vi "Write Roles.vi"(8 "error in (no error)":errorcluster, 10 "Roles":T1, 11 "KickoffEnemyPlayVSS in":refnum<class "KickoffEnemyPlayVSS.lvclass">) -> (0 "error out":errorcluster, 3 "KickoffEnemyPlayVSS out":refnum<class "KickoffEnemyPlayVSS.lvclass">)   [LabVIEW 2020, in "KickoffEnemyPlayVSS.lvclass"]
uses:
  KickoffEnemyPlayVSS.lvclass
  NormalAttackerRoleVSS_class/NormalAttackerRoleVSS.lvclass
  KeeperRoleVSS_class/KeeperRoleVSS.lvclass
  DefenderAreaRoleVSS_class/DefenderAreaRoleVSS.lvclass
  KickoffEnemyPlayVSS.lvclass/KickoffEnemyPlayVSS.ctl
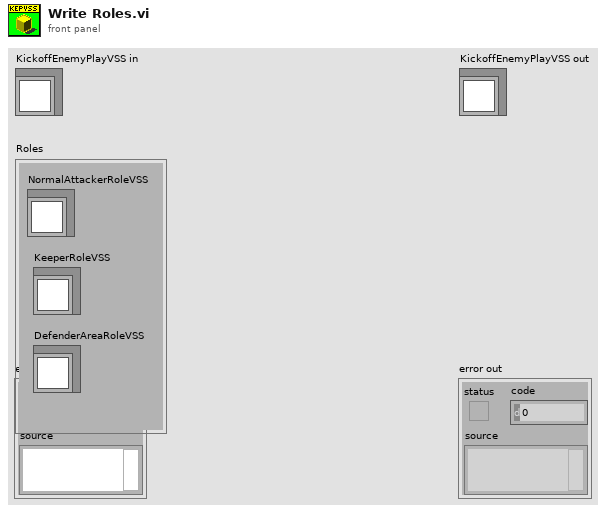
[diagram p1: front panel]
types:
  T1 = cluster{"NormalAttackerRoleVSS":refnum<class "NormalAttackerRoleVSS.lvclass">, "KeeperRoleVSS":refnum<class "KeeperRoleVSS.lvclass">, "DefenderAreaRoleVSS":refnum<class "DefenderAreaRoleVSS.lvclass">}
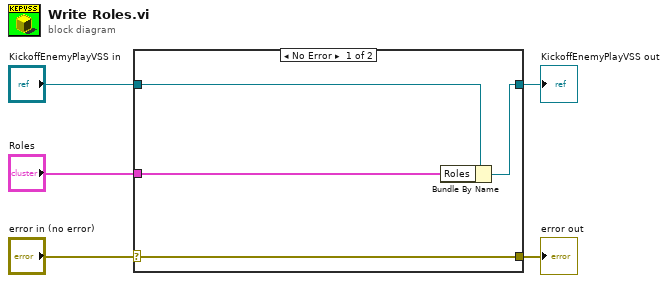
[diagram p0: block diagram]
diagram:
  n1 = case shown="No Error" "error in (no error)" {
    selector: "error in (no error)" -> [w9 w10]
    tunnel: [w9 w10] -> w4
    tunnel: [w7 w11] -> w2
    tunnel: "KickoffEnemyPlayVSS in" -> [w8 w11]
    tunnel: "Roles" -> [w6 _]
    frame No Error {
      n2 = Bundle By Name(cluster=w8, "Roles"=w6) -> (w7:refnum<class "KickoffEnemyPlayVSS.lvclass">)
    }
    frame Error {
    }
  }
  "error out" <- w4
  "KickoffEnemyPlayVSS out" <- w2
